vi "Handle Result.vi"(6 "Prev State":string, 11 "Iteration Result":T1) -> (0 "Abort":bool, 1 "Sequence Mode":T2, 2 "Transition":bool, 3 "State":string)   [LabVIEW 2020, in "VolatusSeq.lvlib" / "Sequence.lvclass"]
uses:
  Sequence.lvclass
  Sequence.lvclass/Sequence.ctl
  Sequence Mode.ctl
  VolatusSeq.lvlib
  Iteration Result.ctl
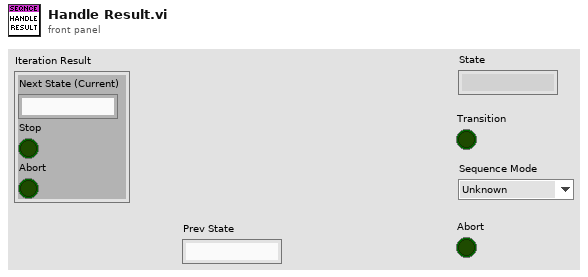
[diagram p1: front panel]
types:
  T1 = typedef "VolatusSeq.lvlib/Iteration Result.ctl" = cluster{"Next State (Current)":string, "Stop":bool, "Abort":bool}
  T2 = typedef "VolatusSeq.lvlib/Sequence Mode.ctl" = enum16{"Unknown", "Loading", "Verifying", "Conflict", "Idle", "Running", "Stopping", "Aborted", "Fault"}
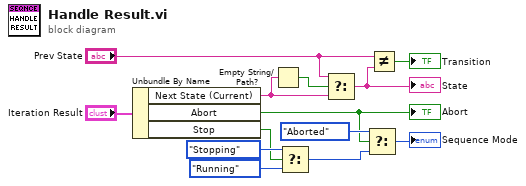
[diagram p0: block diagram]
diagram:
  n1 = Unbundle By Name("Iteration Result") -> ("Next State (Current)"=w9:string, "Abort"=w2:bool, "Stop"=w5:bool)
  "Abort" <- w2
  n2 = Empty String/Path?(string/path=w9) -> (empty?=w13:bool)
  n3 = Select(t=Sequence_Mode."Stopping" ("Sequence Mode"), s=w5, f=Sequence_Mode."Running") -> (s? t:f=w4:T2)
  n4 = Select(t="Prev State", s=w13, f=w9) -> (s? t:f=w12:string)
  "State" <- w12
  n5 = Select(t=Sequence_Mode."Aborted", s=w2, f=w4) -> (s? t:f=→"Sequence Mode":T2)
  n6 = Not Equal?(x="Prev State", y=w12) -> (x != y?=→"Transition":bool)
